vi "System Options.vi"(0 "VISA resource name":refnum<visa-resource-name>, 5 "Display (T: On)":bool=TRUE, 7 "Message (F: Off)":bool, 9 "Message Text (Empty)":string, 11 "error in (no error)":errorcluster) -> (4 "VISA resource name out":refnum<visa-resource-name>, 15 "error out":errorcluster)   [LabVIEW 2013, in "California Instruments iX Series.lvlib"]
doc: "Configure the instrument's front panel display setting."
uses:
  California Instruments iX Series.lvlib
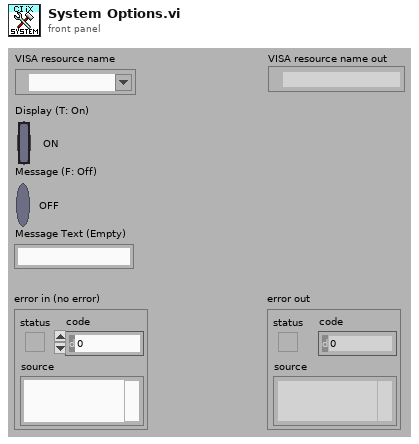
[diagram p1: front panel]
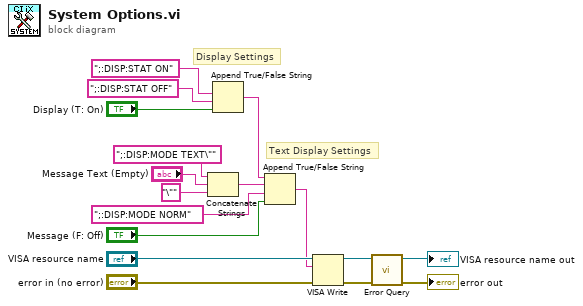
[diagram p0: block diagram]
diagram:
  # "Text Display Settings"
  # "Display Settings"
  n1 = Concatenate Strings(";:DISP:MODE TEXT\"", "Message Text (Empty)", "\"") -> (w6:string)
  n2 = Append True/False String(1:"Display (T: On)", 2:";:DISP:STAT OFF", 3:";:DISP:STAT ON") -> (0:w2:string)  [unwired: 1 in]
  n3 = Append True/False String(1:"Message (F: Off)", 2:";:DISP:MODE NORM", 3:w6, 4:w2) -> (0:w1:string)
  n4 = VISA Write(VISA resource name="VISA resource name", write buffer=w1, error in (no error)="error in (no error)") -> (VISA resource name out=w12:refnum<visa-resource-name>, error out=w11:errorcluster)  [unwired: 1 out]
  n5 = call "Error Query.vi"("error in (no error)"=w11, "VISA resource name"=w12) -> ("error out"=→"error out":errorcluster, "VISA resource name out"=→"VISA resource name out":refnum<visa-resource-name>)  [unwired: 6 in, 2 out]
